vi "c Spark Get Control Frame Period.vi"(8 "error in (no error)":errorcluster, 11 "handle":T1) -> (0 "error out":errorcluster, 2 "function return":i32, 3 "handle out":T1)   [LabVIEW 2023, in "REVLibDriver.lvlib"]
doc: "int c_Spark_GetControlFramePeriod(c_Spark_handle handle);"
uses:
  REVLibDriver.lvlib
  REVLibDriver.dll
  <vilib>/Custom Controls/c_Spark_handle.ctl
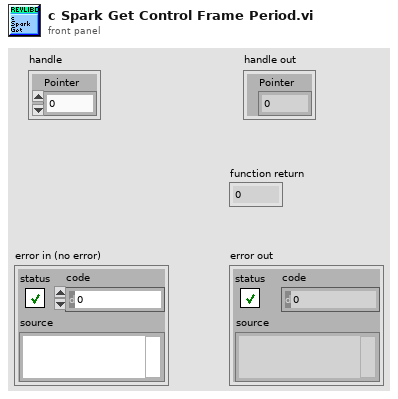
[diagram p1: front panel]
types:
  T1 = typedef "REVLibDriver.lvlib/c_Spark_handle.ctl" = cluster{"Pointer":u32}
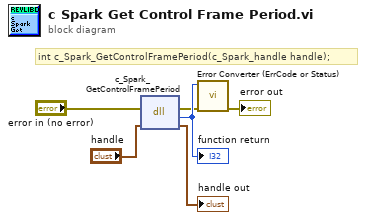
[diagram p0: block diagram]
diagram:
  # "int c_Spark_GetControlFramePeriod(c_Spark_handle handle);"
  n1 = dll-call lib="REVLibDriver.*" fn="c_Spark_GetControlFramePeriod"(error in="error in (no error)", "handle"="handle") -> (error out=w2:errorcluster, w6:i32, "handle"=→"handle out":T1)  [unwired: 2 in, 1 out]
  "function return" <- w6
  n2 = call "Error Converter (ErrCode or Status).vi"("error in (no error)"=w2, "error code"=w6) -> ("error out"=→"error out":errorcluster)  [unwired: 9 in]
